vi "Translate Wheel_Differential.vi"(8 "error in (no error)":errorcluster, 9 "new position":cluster{"x":dbl, "y":dbl}, 10 "wheel index":i32, 11 "differential steering frame in":refnum<class "NI_Robotics_Differential Steering Frame.lvclass">) -> (0 "error out":errorcluster, 3 "differantial steering frame out":refnum<class "NI_Robotics_Differential Steering Frame.lvclass">)   [LabVIEW 2017, in "NI_Robotics_Configure Steering Frame.lvlib"]
uses:
  <vilib>/robotics/Dialog/Configure Steering Frame/NI_Robotics_Configure Steering Frame.lvlib
  <vilib>/robotics/Steering/Differential Steering Frame/NI_Robotics_Differential Steering Frame.lvclass
  c:/Program Files (x86)/National Instruments/LabVIEW 2017/vi.lib/robotics/Steering/Steering Frame/NI_Robotics_Steering Frame.lvclass
  <vilib>/robotics/Steering/Steering Frame/NI_Robotics_Steering Frame.lvclass/NI_Robotics_Steering Frame.ctl
  <vilib>/robotics/Steering/Wheel/NI_Robotics_Wheel.lvclass/NI_Robotics_Wheel.ctl
  <vilib>/robotics/Steering/Differential Steering Frame/NI_Robotics_Differential Steering Frame.lvclass/NI_Robotics_Differential Steering Frame.ctl
  <vilib>/robotics/Steering/Differential Steering Frame/Wheel Separation to Frame Positions.vi
  <vilib>/robotics/Steering/Steering Frame/Reposition Wheels.vi
  <vilib>/robotics/Steering/Wheel/Update Steering to Wheel Frame Transform.vi
  <vilib>/Analysis/coordinate.llb/Wrap Angle.vi
  <vilib>/Analysis/coordinate.llb/Wrap Angle (scalar).vi
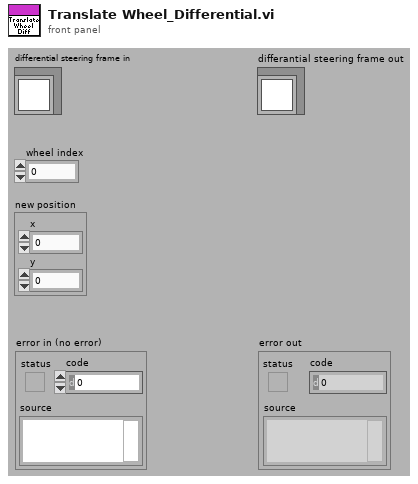
[diagram p1: front panel]
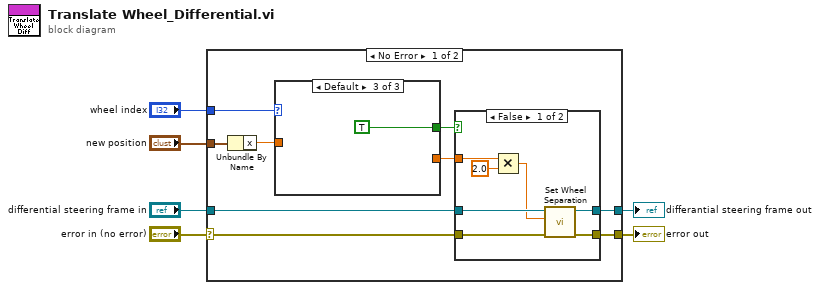
[diagram p0: block diagram]
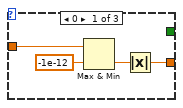
[diagram p3: hidden frame]
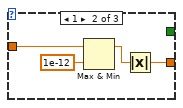
[diagram p4: hidden frame]
diagram:
  n1 = case shown="No Error" "error in (no error)" {
    selector: "error in (no error)" -> [w10 w34]
    tunnel: "differential steering frame in" -> [w11 w35]
    tunnel: [w9 w35] -> w4
    tunnel: [w8 w34] -> w3
    tunnel: "wheel index" -> [w15 _]
    tunnel: "new position" -> [w14 _]
    frame No Error {
      n2 = Unbundle By Name(w14) -> ("x"=w13:dbl)
      n3 = case shown="Default" w15 {
        tunnel: w13 -> [w28 w32 _]
        tunnel: [w25 w30 _] -> w12
        tunnel: [_ _ TRUE] -> w7
        frame 0 {
          n4 = Max & Min(x=w28, y=-1e-12) -> (min(x,y)=w26:dbl)  [unwired: 1 out]
          n5 = Absolute Value(x=w26) -> (abs(x)=w25:dbl)
        }
        frame 1 {
          n6 = Max & Min(x=w32, y=1e-12) -> (max(x,y)=w29:dbl)  [unwired: 1 out]
          n7 = Absolute Value(x=w29) -> (abs(x)=w30:dbl)
        }
        frame Default {
        }
      }
      n8 = case shown="False" w7 {
        tunnel: w12 -> [w22 _]
        tunnel: w11 -> [w20 w24]
        tunnel: w10 -> [w18 w23]
        tunnel: [w17 w24] -> w9
        tunnel: [w16 w23] -> w8
        frame False {
          n9 = Multiply(x=w22, y=2.0) -> (x*y=w19:dbl)
          n10 = call <vilib>:"Set Wheel Separation.vi"("error in (no error)"=w18, "wheel separation"=w19, "differential steering frame in"=w20) -> ("error out"=w16:errorcluster, "differential steering frame out"=w17:refnum<class "NI_Robotics_Differential Steering Frame.lvclass">)  [unwired: 7 in]
        }
        frame True {
        }
      }
    }
    frame Error {
    }
  }
  "differantial steering frame out" <- w4
  "error out" <- w3
